vi "AdjustThomsonTimings.vi"(10 "Hold off Guess":dbl, 11 "Input Trigger Data":T3) -> (3 "Output Trigger Data":T3)   [LabVIEW 2016]
uses:
  Ctrl_Signal.ctl
  Ctrl_Signal_Map.ctl
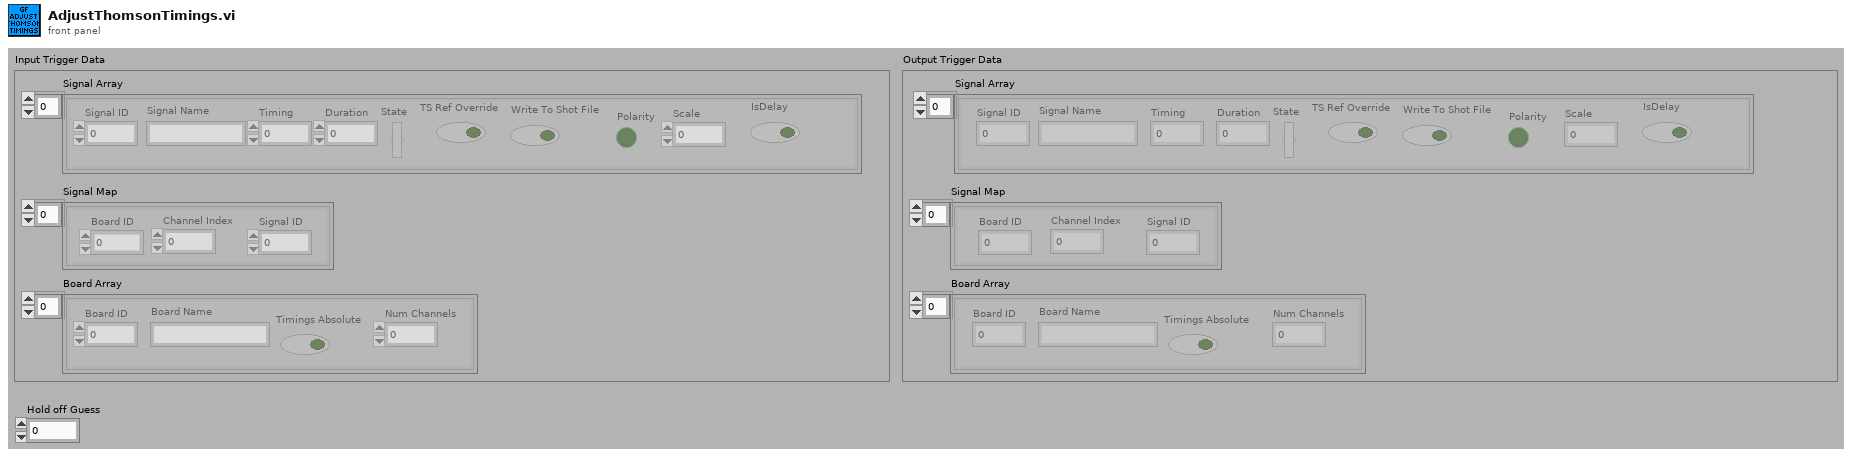
[diagram p1: front panel]
types:
  T1 = typedef "Ctrl_Signal.ctl" = cluster{"Signal Name":string, "Timing":dbl, "Duration":dbl, "State":bool, "TS Ref Override":bool, "Write To Shot File":bool, "Polarity":bool, "Signal ID":dbl, "Scale":dbl, "IsDelay":bool}
  T2 = typedef "Ctrl_Signal_Map.ctl" = cluster{"Channel Index":dbl, "Board ID":dbl, "Signal ID":dbl}
  T3 = cluster{"Signal Array":T1[], "Signal Map":T2[], "Board Array":cluster{"Board ID":dbl, "Board Name":string, "Timings Absolute":bool, "Num Channels":dbl}[]}
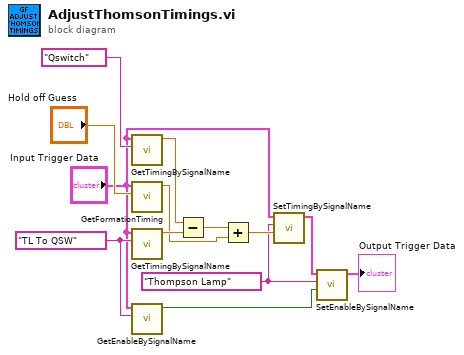
[diagram p0: block diagram]
diagram:
  w2 = "Thompson Lamp" ("Signal Name")
  w7 = "TL To QSW" ("Signal Name")
  n1 = call "GetTimingBySignalName.vi"("Signal Name"="Qswitch", "Trigger Data"="Input Trigger Data") -> ("Timing"=w11:dbl)  [unwired: 9 in]
  n2 = call "GetFormationTiming.vi"("Hold off Guess"="Hold off Guess", "Trigger Data"="Input Trigger Data") -> ("Formation Timing"=w8:dbl)  [unwired: 9 in]
  n3 = call "GetTimingBySignalName.vi"("Signal Name"=w7, "Trigger Data"="Input Trigger Data") -> ("Timing"=w10:dbl)  [unwired: 9 in]
  n4 = call "GetEnableBySignalName.vi"("Signal Name"=w7, "Trigger Data"="Input Trigger Data") -> ("Signal Enabled"=w1:bool)  [unwired: 9 in]
  n5 = Subtract(x=w11, y=w10) -> (x-y=w9:dbl)
  n6 = Add(x=w9, y=w8) -> (x+y=w3:dbl)
  n7 = call "SetTimingBySignalName.vi"("Timing"=w3, "Signal Name"=w2, "Trigger Data Input"="Input Trigger Data") -> ("Trigger Data Output"=w6:T3)  [unwired: 8 in]
  n8 = call "SetEnableBySignalName.vi"("State"=w1, "Signal Name"=w2, "Trigger Data Input"=w6) -> ("Trigger Data Output"=→"Output Trigger Data":T3)  [unwired: 8 in]
